vi "Port Checking Error String-LabJack.vi"(2 "Ch Index":i32, 3 "Port":string) -> (0 "error out":errorcluster)   [LabVIEW 2017]
uses:
  Globals/Meas_global.vi
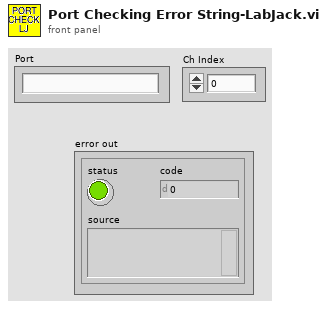
[diagram p1: front panel]
types:
  T1 = typedef "Analysis_info_cluster.ctl" = cluster{"Colour":u32, "Inst type":T2, "Inst name":string, "Symbol":string, "Code name":string, "Extra Info":string, "Inst Array":T3, "Extra Titles":string[], "Extra Values":string[], "U":dbl, "u^2":dbl, "u^3":dbl, "u^4":dbl, "Skew_u":dbl, "Kurt_u":dbl, "Sd Error in Mean":dbl, "% u'/U":dbl, "X":dbl, "Y":dbl, "Z":dbl, "Timescale integral Estimate":dbl, "Sd Error in Variance":dbl, "Calib File":path, "Calib Constants":dbl[], "Output Position":bool, "Full Stats":bool, "Av Sampling Rate":dbl, "Av No of Samples":dbl, "Total Meas Time (s)":dbl, "ADAM Ch Name":string, "Max value":dbl, "Min value":dbl, "Req Sample Rate Hz":dbl, "Sync Delay Time (s)":dbl, "Ch No":i16, "Device":string, "Use Latest Calib":bool, "Port":string, "Metadata Ch Names":string[], "Metadata Ch Values":string[]}
  T2 = typedef "Inst_type.ctl" = enum16{"Propeller anemometer", "Raw voltage", "Pressure Transducer", "Pitot-static tube", "Preston tube", "Hot wire", "Cross wire 1", "Cross wire 2", "Generic Linear", "Generic Polynomial", "Generic BackPoly", "Fast FID", "Thermocouple", "Cold wire", "Pulsed Wire", "LDA Vel", "LDA Tran time", "LDA Arr time", "Microphone"}
  T3 = typedef "Instrument_Array.ctl" = enum16{"PWA", "LDA", "Analogue"}
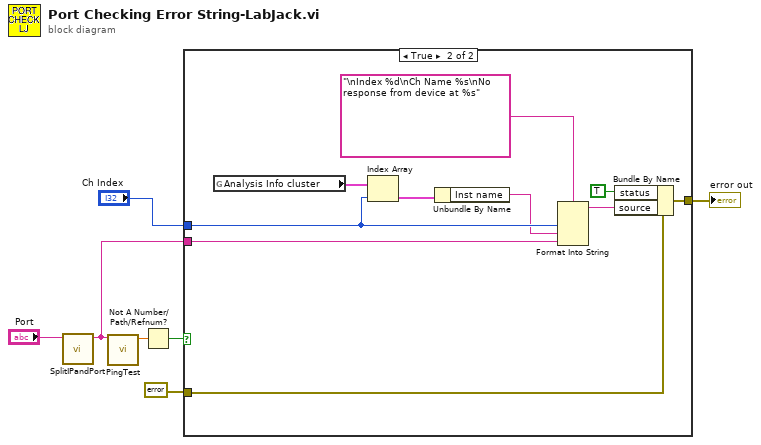
[diagram p0: block diagram]
diagram:
  n1 = call "SplitIPandPort.vi"("IP:Port"="Port") -> ("IP"=w1:string)  [unwired: 9 in, 1 out]
  n2 = call "PingTest.vi"("IP Address"=w1) -> ("Reading"=w4:dbl)  [unwired: 9 in, 1 out]
  n3 = Not A Number/Path/Refnum?(number/path/refnum=w4) -> (NaN/Path/Refnum?=w3:bool)
  n4 = case shown="True" w3 {
    tunnel: "Ch Index" -> [_ w16]
    tunnel: w1 -> [_ w9]
    tunnel: [w8 w12] -> w5
    tunnel: errorcluster {"status"=FALSE, "code"=0, "source"=""} ("error out") -> [w8 w13]
    frame False {
    }
    frame True {
      n5 = global read "Meas_global.vi" "Analysis Info cluster"() -> (w17:T1[])
      n6 = Index Array(array=w17, index=w16) -> (element=w15:T1)
      n7 = Unbundle By Name(w15) -> ("Inst name"=w14:string)
      n8 = Format Into String(format string="\nIndex %d\nCh Name %s\nNo response from device at %s", w16, w14, w9) -> (resulting string=w10:string)  [unwired: 2 in, 1 out]
      n9 = Bundle By Name(cluster=w13, "status"=TRUE, "source"=w10) -> (w12:errorcluster)
    }
  }
  "error out" <- w5
